vi "Demo - Transfer Modes.vi"() -> ()   [LabVIEW 2013, in "GOLPI library.lvlib"]
doc: "Shows advantages and disadvantages of different transfer modes of data between GNU Octave and LabVIEW.\n\n---\nGOLPI works only with lv_proc.dll library, which is part of vipm package or should be delivered together with packed library. Placement of this dll is selected in terminal of Start GNU Octave.vi."
uses:
  GOLPI library.lvlib
  Private/Get Variable - polymorph parts/Get Struct.vi
  Private/Set Variable - polymorph parts/Set 1D Array Double.vi
  Private/Get Variable - polymorph parts/Get 1D Array Double.vi
panel:
  in  "stop":bool
  out "Bitstream mode transfer time (ms):":u32[](array[numeric])
  out "Temporary file mode transfer time (ms):":u32[](array[numeric])
  out "Normal mode transfer time (ms):":u32[](array[numeric])
  in  "Test vector sizes":i32[](array[numeric])=[2, 20000]
  out "LabVIEW Cluster":T1
  in  "octave exe file or directory":path=path "C:/Octave/Octave-4.0.0/bin"
  out "exit code of GNU\nOctave process:":i32
  out "error out":errorcluster
  in  "working directory":path=path "C:/"
  # "1, start up"
  # "For Bitstream transsfer mode and for transfer of structures GNU Octave\npackage golpi is required. VIs will try to install it, if not found, you will be\nasked to find positiion of the fiel with the package.\n(golpi-X.X.X.tar.gz, where X is number)"
  # "GNU Octave is started, executable is placed in this directory:"
  # "Working directory is set to:"
  # "2, transfer mode speed comparison"
  # "Two vectors, small and large one, with number of elements                                          are prepared in LabVIEW."
  # "Normal tranfer mode: data are sent into GNU Octave using commands. Data are sent\nto LabVIEW  in such a way content of variables is printed to console and parsed by\nLabVIEW.\n\nTemporary file transfer mode: a temporary file in version 4 .mat format with the\ndata is created. Both GNU Octave and GOLPI can read the format directly.\n\nBitstream transfer mode: data are sent into GNU Octave using commands. Back to LabVIEW\ndata are converted into special series of bytes, bytes are printed to console and parsed\nby LabVIEW."
  # "These vectors are transfered to GNU Octave and back. Transfer times for different transfer modes are:"
  # "One can see the normal mode is fast for small data and slow for large ones. Using temporary file gives similar transfer \ntime, almost independent on the size of data. Bitstream mode gives faster results than normal mode, but output in \nconsole is not human readable."
  # "3, transfer of GNU Octave structure to LabVIEW cluster"
  # "GNU Octave structures can be transfered to LabVIEW cluster. Cluster must contain elements of the same name\nas structure fields and same data type. Structure can have extra fields and cluster can contain extra elements."
  # "In this example following structure is transfered to following cluster."
  # "GNU Octave structure\n\ns.num=5\ns.str=\"test\"\ns.mat = magic(3)\ns.not_in_cluster=-5"
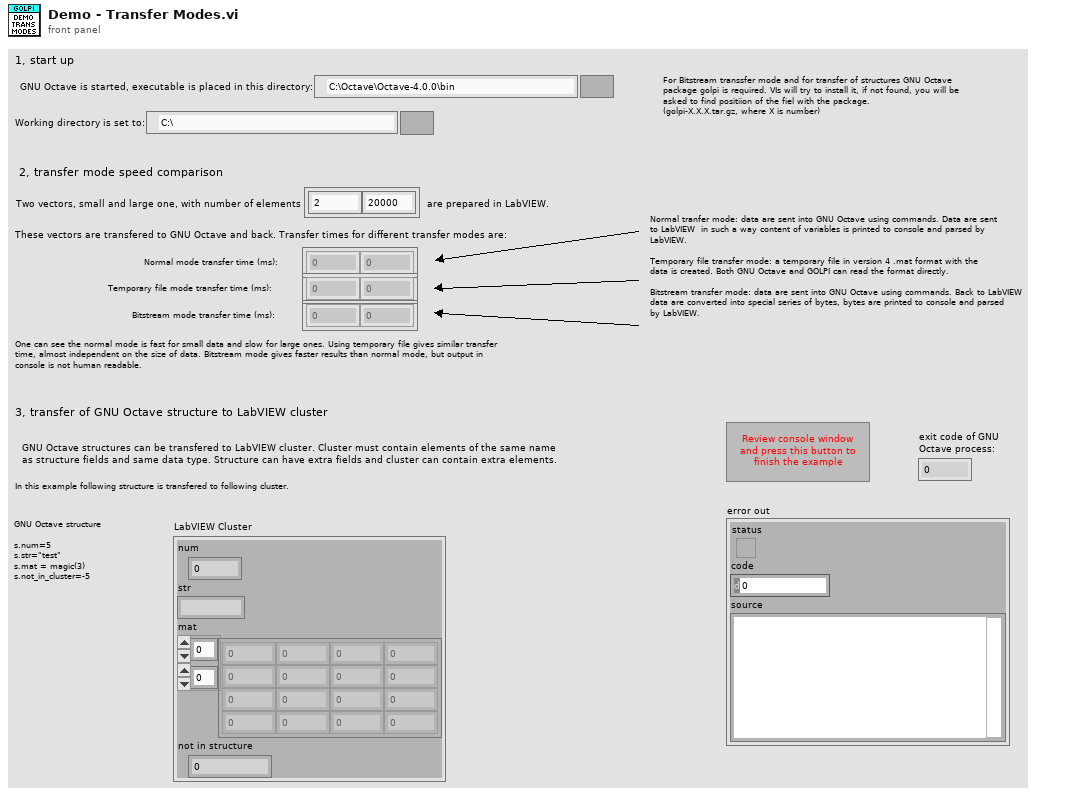
[diagram p1: front panel]
types:
  T1 = cluster{"num":dbl, "str":string, "mat":dbl[][], "not in structure":dbl}
  T2 = typedef "GOLPI library.lvlib/GOLPI reference Type Def.ctl" = cluster{"pipe handle":T3, "fast read timeout [ms]":u32, "fast read settle time [ms]":u32, "fast read to multiple [ms]":u32, "max elements per input line":u32, "slow read timeout [ms]":u32, "stdin double format specifier":string, "max elements per stdout output column":u32, "console mode bitstream":bool, "bitstream first read timeout [ms]":u32, "bitstream read timeout [ms]":u32, "struct transfer possible":bool}
  T3 = typedef "LV Process library.lvlib/Pipe Handle.ctl" = cluster{"lv_proc.dll file path":path, "process instance handle":u32[], "debug mode":bool, "debug data":cluster{"time":timestamp, "stdin":bool, "data":string}[]}
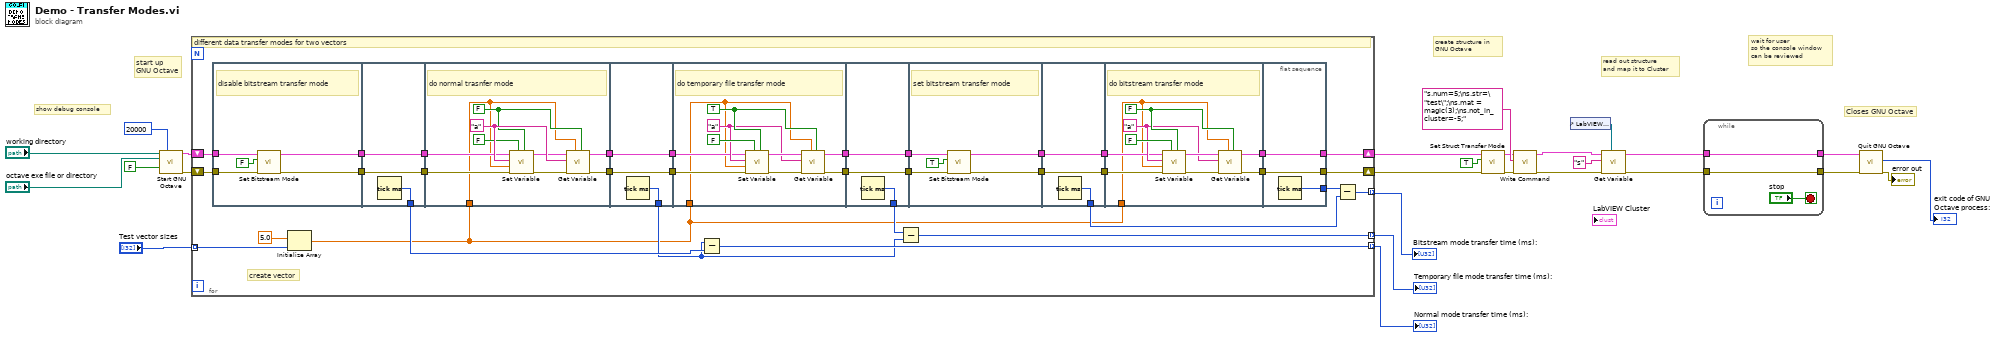
[diagram p0: block diagram]
diagram:
  # "wait for user\nso the console window\ncan be reviewed"
  # "read out structure\nand map it to Cluster"
  # "create structure in\nGNU Octave"
  # "start up\nGNU Octave"
  # "show debug console"
  # "Closes GNU Octave"
  n1 = call "Start GNU Octave.vi"("working directory"="working directory", "full start timeout [ms] (20000)"=u32 20000 ("Full start timeout [ms] (5000)"), "octave exe file or directory"="octave exe file or directory", "hide debug console (T)"=FALSE) -> ("GOLPI ref. out"=w20:T2, "error out"=w19:errorcluster)  [unwired: 8 in, 2 out]
  n2 = for {
    tunnel: "Test vector sizes" -> [w42] mode=indexing
    tunnel: [w40] -> w17 mode=indexing
    tunnel: [w35] -> w16 mode=indexing
    tunnel: [w33] -> w15 mode=indexing
    shift-right: [w30] -> w13
    shift-left: w19 -> [w38]
    shift-right: [w29] -> w14
    shift-left: w20 -> [w39]
    # "create vector"
    # "different data transfer modes for two vectors"
    n3 = flat-sequence {
      tunnel: w38 -> [w62]
      tunnel: w39 -> [w63]
      tunnel: [w61] -> w28
      tunnel: [w60] -> w27
      tunnel: [w67] -> w41
      tunnel: [w66] -> w59
      tunnel: [w65] -> w58
      tunnel: w28 -> [w66]
      tunnel: w27 -> [w65]
      tunnel: w59 -> [w76]
      tunnel: w58 -> [w75]
      tunnel: [w71] -> w57
      tunnel: [w72] -> w56
      tunnel: w32 -> [w68]
      tunnel: w57 -> [w80]
      tunnel: w56 -> [w79]
      tunnel: [w80] -> w55
      tunnel: [w79] -> w54
      tunnel: [w78] -> w36
      tunnel: w55 -> [w85]
      tunnel: w54 -> [w84]
      tunnel: [w83] -> w53
      tunnel: [w82] -> w52
      tunnel: w32 -> [w81]
      tunnel: w53 -> [w93]
      tunnel: [w91] -> w37
      tunnel: w52 -> [w92]
      tunnel: [w93] -> w51
      tunnel: [w92] -> w50
      tunnel: w51 -> [w98]
      tunnel: w50 -> [w95]
      tunnel: [w97] -> w49
      tunnel: [w96] -> w48
      tunnel: w49 -> [w101]
      tunnel: w48 -> [w100]
      tunnel: [w101] -> w47
      tunnel: [w100] -> w46
      tunnel: [w99] -> w34
      tunnel: w47 -> [w106]
      tunnel: w46 -> [w105]
      tunnel: [w104] -> w45
      tunnel: [w103] -> w44
      tunnel: w32 -> [w102]
      tunnel: w45 -> [w112]
      tunnel: w44 -> [w113]
      tunnel: [w114] -> w31
      tunnel: [w113] -> w30
      tunnel: [w112] -> w29
      frame #0 {
        # "disable bitstream transfer mode"
        n4 = call "Set Bitstream Mode.vi"("error in"=w62, "Bitstream mode (F)"=FALSE, "GOLPI ref. in"=w63) -> ("error out"=w60:errorcluster, "GOLPI ref. out"=w61:T2)  [unwired: 7 in]
      }
      frame #1 {
        n5 = Tick Count (ms)() -> (millisecond timer value=w67:u32)
      }
      frame #2 {
        w70 = FALSE ("use temporary file? (F)")
        w77 = "a" ("variable name")
        # "do normal trasnfer mode"
        n6 = call-poly "Set Variable.vi"("use temporary file? (F)"=w70, "column vector?"=FALSE, "error in"=w75, "value"=w68, "variable name"=w77, "GOLPI ref. in"=w76) -> ("error out"=w73:errorcluster, "GOLPI ref. out"=w74:T2)  [unwired: 4 in]
        n7 = call-poly "Get Variable.vi"("use temporary file? (F)"=w70, "data type of variable"=w68, "error in"=w73, "variable name"=w77, "GOLPI ref. in"=w74) -> ("error out"=w72:errorcluster, "GOLPI ref. out"=w71:T2)  [unwired: 4 in, 1 out]
      }
      frame #3 {
        n8 = Tick Count (ms)() -> (millisecond timer value=w78:u32)
      }
      frame #4 {
        w89 = TRUE ("use temporary file? (F)")
        w86 = "a" ("variable name")
        # "do temporary file transfer mode"
        n9 = call-poly "Set Variable.vi"("use temporary file? (F)"=w89, "column vector?"=FALSE, "error in"=w84, "value"=w81, "variable name"=w86, "GOLPI ref. in"=w85) -> ("error out"=w88:errorcluster, "GOLPI ref. out"=w87:T2)  [unwired: 4 in]
        n10 = call-poly "Get Variable.vi"("use temporary file? (F)"=w89, "data type of variable"=w81, "error in"=w88, "variable name"=w86, "GOLPI ref. in"=w87) -> ("error out"=w82:errorcluster, "GOLPI ref. out"=w83:T2)  [unwired: 4 in, 1 out]
      }
      frame #5 {
        n11 = Tick Count (ms)() -> (millisecond timer value=w91:u32)
      }
      frame #6 {
        # "set bitstream transfer mode"
        n12 = call "Set Bitstream Mode.vi"("error in"=w95, "Bitstream mode (F)"=TRUE, "GOLPI ref. in"=w98) -> ("error out"=w96:errorcluster, "GOLPI ref. out"=w97:T2)  [unwired: 7 in]
      }
      frame #7 {
        n13 = Tick Count (ms)() -> (millisecond timer value=w99:u32)
      }
      frame #8 {
        w110 = FALSE ("use temporary file? (F)")
        w107 = "a" ("variable name")
        # "do bitstream transfer mode"
        n14 = call-poly "Set Variable.vi"("use temporary file? (F)"=w110, "column vector?"=FALSE, "error in"=w105, "value"=w102, "variable name"=w107, "GOLPI ref. in"=w106) -> ("error out"=w109:errorcluster, "GOLPI ref. out"=w108:T2)  [unwired: 4 in]
        n15 = call-poly "Get Variable.vi"("use temporary file? (F)"=w110, "data type of variable"=w102, "error in"=w109, "variable name"=w107, "GOLPI ref. in"=w108) -> ("error out"=w103:errorcluster, "GOLPI ref. out"=w104:T2)  [unwired: 4 in, 1 out]
      }
      frame #9 {
        n16 = Tick Count (ms)() -> (millisecond timer value=w114:u32)
      }
    }
    n17 = Initialize Array(5.0 ("element"), w42) -> (w32:dbl[])
    n18 = Subtract(x=w36, y=w41) -> (x-y=w40:u32)
    n19 = Subtract(x=w37, y=w36) -> (x-y=w35:u32)
    n20 = Subtract(x=w31, y=w34) -> (x-y=w33:u32)
  }
  "Normal mode transfer time (ms):" <- w17
  "Temporary file mode transfer time (ms):" <- w16
  "Bitstream mode transfer time (ms):" <- w15
  n21 = call "Set Struct Transfer Mode.vi"("error in"=w13, "Allow struct tranfer (False)"=TRUE, "GOLPI ref. in"=w14) -> ("error out"=w10:errorcluster, "GOLPI ref. out"=w11:T2)  [unwired: 6 in, 1 out]
  n22 = call "Write Command.vi"("error in"=w10, "command"="s.num=5;\ns.str=\"test\";\ns.mat = magic(3);\ns.not_in_cluster=-5;", "GOLPI ref. in"=w11) -> ("error out"=w8:errorcluster, "GOLPI ref. out"=w9:T2)  [unwired: 7 in]
  n23 = control-ref of="LabVIEW Cluster"() -> (w7:refnum<vi>)
  n24 = call-poly "Get Variable.vi"("cluster ref (empty)"=w7, "error in"=w8, "variable"="s", "GOLPI ref in"=w9) -> ("error out"=w3:errorcluster, "GOLPI ref. out"=w1:T2)  [unwired: 5 in, 1 out]
  n25 = while {
    tunnel: [w117] -> w4
    tunnel: w3 -> [w117]
    tunnel: [w115] -> w2
    tunnel: w1 -> [w115]
    stop <- "stop" stop-if-true
  }
  n26 = call "Quit GNU Octave.vi"("error in"=w4, "GOLPI ref. in"=w2) -> ("error out"=→"error out":errorcluster, "exit code"=→"exit code of GNU\nOctave process:":i32)  [unwired: 8 in]
